vi "Begin.vi"(11 "Image Size":T1=enum."160x120") -> (0 "error out":errorcluster)   [LabVIEW 2012]
doc: "Called before other user functions, this VI is expected to open initial I/O refnums, load in file data, and do all program initialization. Notice that the <B>error out</B> terminal is simply used for data flow. Wiring it to other structures or subVIs ensures that this VI runs first."
uses:
  <vilib>/Rock Robotics/WPI/Camera/WPI_CameraImageSize.ctl
  <vilib>/Rock Robotics/SystemInterfaces/DIO/FPGA_DIOPWMChannel.ctl
  <vilib>/Rock Robotics/WPI/Camera/WPI_CameraWhite Balance Values.ctl
  <vilib>/Rock Robotics/WPI/Camera/WPI_CameraExposure Values.ctl
  <vilib>/Rock Robotics/WPI/Camera/WPI_CameraFrameRate.ctl
  <vilib>/Rock Robotics/WPI/DriverStation/WPI_DriverStationRobotMode2.ctl
  <vilib>/Rock Robotics/WPI/Joystick/WPI_JoystickDeviceEnum.ctl
  <vilib>/Rock Robotics/WPI/Solenoid/WPI_SolenoidChannel.ctl
  <vilib>/Rock Robotics/SystemInterfaces/DIO/FPGA_DIORelayChannel.ctl
  <vilib>/Rock Robotics/SystemInterfaces/DIO/FPGA_DIOChannel.ctl
  <vilib>/Rock Robotics/WPI/SafetyOutput/WPI_SafetyOutputConfigMenu.ctl
  <vilib>/Rock Robotics/WPI/RobotDrive/WPI_RobotDriveOpen2MotorWithJaguar.vi
  Robot Global Data.vi
  <vilib>/Rock Robotics/WPI/MotorControl/WPI_MotorControlOpen Jaguar.vi
  <vilib>/Rock Robotics/WPI/Solenoid/WPI_SolenoidOpenDouble.vi
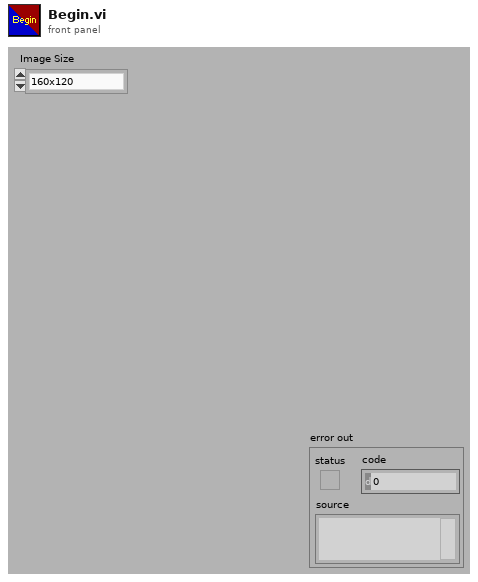
[diagram p1: front panel]
types:
  T1 = typedef "WPI_CameraImageSize.ctl" = enum16{"640x480", "320x240", "160x120"}
  T2 = typedef "WPI_SafetyOutputConfigMenu.ctl" = enum16{"Enable", "Disable"}
  T3 = typedef "FPGA_DIOPWMChannel.ctl" = enum8{"PWM 1", "PWM 2", "PWM 3", "PWM 4", "PWM 5", "PWM 6", "PWM 7", "PWM 8", "PWM 9", "PWM 10", "Invalid"}
  T4 = typedef "FPGA_DIORelayChannel.ctl" = enum8{"Relay 1", "Relay 2", "Relay 3", "Relay 4", "Relay 5", "Relay 6", "Relay 7", "Relay 8", "Invalid"}
  T5 = typedef "FPGA_DIOChannel.ctl" = enum8{"DIO 1", "DIO 2", "DIO 3", "DIO 4", "DIO 5", "DIO 6", "DIO 7", "DIO 8", "DIO 9", "DIO 10", "DIO 11", "DIO 12", "DIO 13", "DIO 14", "Invalid"}
  T6 = typedef "WPI_SolenoidChannel.ctl" = enum8{"Solenoid 1", "Solenoid 2", "Solenoid 3", "Solenoid 4", "Solenoid 5", "Solenoid 6", "Solenoid 7", "Solenoid 8", "Invalid"}
  T7 = typedef "WPI_JoystickDeviceEnum.ctl" = enum16{"USB 1", "USB 2", "USB 3", "USB 4", "Kinect 1", "Kinect 2"}
  T8 = typedef "WPI_DriverStationRobotMode2.ctl" = enum16{"Autonomous Disabled", "Autonomous Enabled", "Teleop Disabled", "Teleop Enabled", "Timeout", "Finish", "Test Disabled", "Test Enabled"}
  T9 = typedef "WPI_CameraFrameRate.ctl" = u32
  T10 = typedef "WPI_CameraExposure Values.ctl" = enum16{"Auto", "Flicker-free 50 Hz", "Flicker-free 60 Hz", "Hold current"}
  T11 = typedef "WPI_CameraWhite Balance Values.ctl" = enum16{"Auto", "Fixed indoor", "Fixed outdoor 1", "Fixed outdoor 2", "Fixed fluorescent 1", "Fixed fluorescent 2", "Hold current"}
  T12 = typedef "WPI_DigitalInputDevRef.ctl" = cluster{"DevStatus":errorcluster, "DIO Channel":T5, "Digital Module":T13}
  T13 = typedef "FPGA_TypedefDigitalModule.ctl" = enum16{"Digital Module 1", "Digital Module 2"}
  T14 = typedef "WPI_SolenoidDevRef.ctl" = cluster{"DevStatus":errorcluster, "Solenoid Module":T15, "Forward Solenoid Channel":T6, "Reverse Solenoid Channel":T6}
  T15 = typedef "FPGA_TypedefSolenoidModule.ctl" = enum16{"Solenoid Module 1", "Solenoid Module 2"}
  T16 = typedef "WPI_CameraDevRef.ctl" = cluster{"Camera Address":string, "CameraStatus":errorcluster, "Acquire Image Notifier":refnum<notifier>}
  T17 = typedef "WPI_JoystickDevRef.ctl" = cluster{"Device":T7}
  T18 = typedef "WPI_RobotDriveDevRef.ctl" = cluster{"DevStatus":errorcluster, "Motors[]":T19[], "Square Inputs":bool, "Max Output":dbl, "Isochronous":bool}
  T19 = typedef "WPI_MotorControlDeviceRef.ctl" = cluster{"DeviceStatus":errorcluster, "Type":enum16{"PWM", "CAN"}, "PWM":cluster{"Digital Module":T13, "PWM Channel":T3, "DeadBand":T20}, "CAN":cluster{"Device Number":u8, "Control Mode":T21, "Semaphore":T22, "Max Vout":dbl}, "Invert":bool, "TransformRef":T23, "InvTransformRef":T23}
  T20 = typedef "WPI_PWMDeadband.ctl" = cluster{"Name":string, "maxPositivePwm":i32, "minPositivePwm":i32, "centerPwm":i32, "maxNegativePwm":i32, "minNegativePwm":i32, "angularRange":u16}
  T21 = typedef "WPI_CANJaguar_ControlMode.ctl" = enum8{"Percent VBus", "Current", "Speed", "Position", "Voltage"}
  T22 = typedef "Semaphore RefNum" = refnum<k1>
  T23 = typedef "WPI_PWMTransform_ConPane.ctl" = refnum<vi>
  T24 = typedef "WPI_RelayDevRef.ctl" = cluster{"DevStatus":errorcluster, "Relay Channel":T4, "Digital Module":T13, "Relay Direction":T25}
  T25 = typedef "WPI_RelayDirection.ctl" = enum16{"Both directions", "Forward only", "Reverse only"}
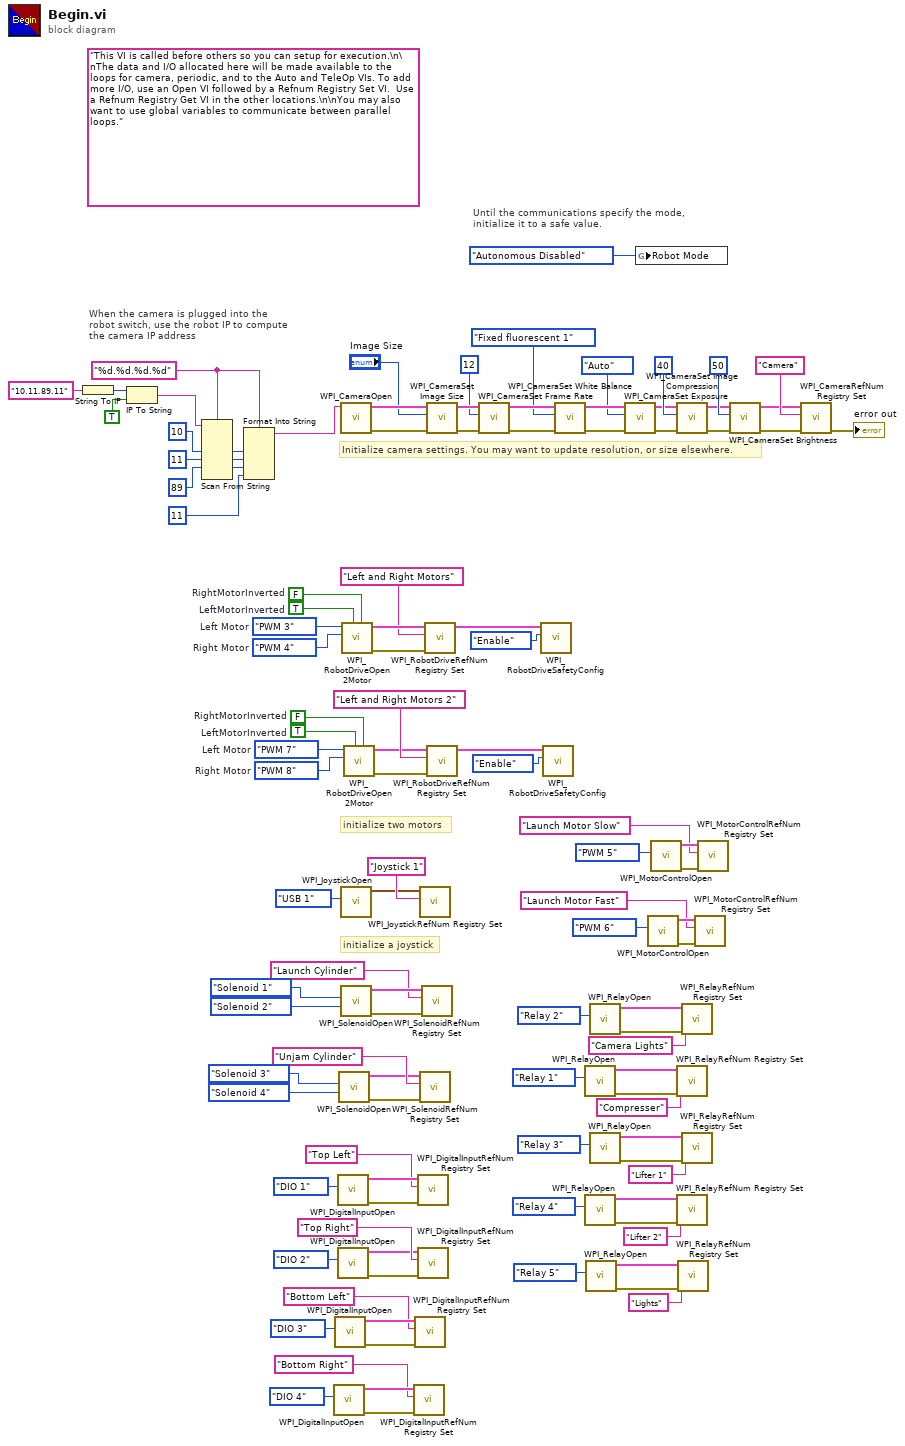
[diagram p0: block diagram]
diagram:
  w7 = FPGA_DIOPWMChannel."PWM 8"  # Right Motor
  w6 = FPGA_DIOPWMChannel."PWM 7"  # Left Motor
  w2 = TRUE  # LeftMotorInverted
  w1 = FALSE  # RightMotorInverted
  w76 = "%d.%d.%d.%d" ("format string")
  (unwired) "This VI is called before others so you can setup for execution.\n\nThe data and I/O allocated here will be made available to the loops for camera, periodic, and to the Auto and TeleOp VIs. To add more I/O, use an Open VI followed by a Refnum Registry Set VI.  Use a Refnum Registry Get VI in the other locations.\n\nYou may also want to use global variables to communicate between parallel loops."
  w87 = FPGA_DIOPWMChannel."PWM 4"  # Right Motor
  w88 = FPGA_DIOPWMChannel."PWM 3"  # Left Motor
  w110 = TRUE  # LeftMotorInverted
  w111 = FALSE  # RightMotorInverted
  # "initialize a joystick"
  # "Until the communications specify the mode,\ninitialize it to a safe value."
  # "When the camera is plugged into the\nrobot switch, use the robot IP to compute\nthe camera IP address"
  # "initialize two motors"
  # "Initialize camera settings. You may want to update resolution, or size elsewhere."
  n1 = String To IP(1:"10.11.89.11" ("name")) -> (0:w83:u32)
  n2 = IP To String(1:TRUE ("dot notation? (F)"), 2:w83) -> (0:w81:string)
  n3 = Scan From String(format string=w76, input string=w81, default 1=10 ("default value 1"), default 2=11 ("default value 2"), default 3=89 ("default value 3")) -> (output 1=w80:i32, output 2=w79:i32, output 3=w78:i32)  [unwired: 4 in, 3 out]
  n4 = Format Into String(format string=w76, w80, w79, w78, 11 ("Compression")) -> (resulting string=w72:string)  [unwired: 2 in, 1 out]
  n5 = call <vilib>:"WPI_DigitalInputOpen.vi"("DIO Channel"=FPGA_DIOChannel."DIO 4") -> ("error out"=w16:errorcluster, "DigitalInputDevRef"=w17:T12)  [unwired: 9 in]
  n6 = call <vilib>:"WPI_DigitalInputOpen.vi"("DIO Channel"=FPGA_DIOChannel."DIO 3") -> ("error out"=w21:errorcluster, "DigitalInputDevRef"=w20:T12)  [unwired: 9 in]
  n7 = call <vilib>:"WPI_DigitalInputOpen.vi"("DIO Channel"=FPGA_DIOChannel."DIO 1") -> ("error out"=w29:errorcluster, "DigitalInputDevRef"=w28:T12)  [unwired: 9 in]
  n8 = call <vilib>:"WPI_DigitalInputOpen.vi"("DIO Channel"=FPGA_DIOChannel."DIO 2") -> ("error out"=w22:errorcluster, "DigitalInputDevRef"=w23:T12)  [unwired: 9 in]
  n9 = call-poly <vilib>:"WPI_SolenoidOpen.vi"("Reverse Solenoid Channel"=WPI_SolenoidChannel."Solenoid 4", "Forward Solenoid Channel"=WPI_SolenoidChannel."Solenoid 3") -> ("error out"=w42:errorcluster, "SolenoidDevRef"=w43:T14)  [unwired: 8 in]
  n10 = call <vilib>:"WPI_CameraOpen.vi"("Camera Address"=w72) -> ("error out"=w97:errorcluster, "CameraDevRef"=w98:T16)  [unwired: 1 in, 8 out]
  n11 = call <vilib>:"WPI_JoystickOpen.vi"("JoystickDevice"=WPI_JoystickDeviceEnum."USB 1") -> ("JoystickDevRef"=w70:T17)  [unwired: 10 in]
  n12 = call-poly <vilib>:"WPI_SolenoidOpen.vi"("Reverse Solenoid Channel"=WPI_SolenoidChannel."Solenoid 2", "Forward Solenoid Channel"=WPI_SolenoidChannel."Solenoid 1") -> ("error out"=w55:errorcluster, "SolenoidDevRef"=w54:T14)  [unwired: 8 in]
  n13 = call-poly <vilib>:"WPI_RobotDriveOpen2Motor.vi"("Right Motor Inverted"=w111, "Left Motor Inverted"=w110, "Right Motor"=w87, "Left Motor"=w88) -> ("error out"=w106:errorcluster, "RobotDriveDevRef"=w108:T18)  [unwired: 1 in, 5 out]
  n14 = call-poly <vilib>:"WPI_RobotDriveOpen2Motor.vi"("Right Motor Inverted"=w1, "Left Motor Inverted"=w2, "Right Motor"=w7, "Left Motor"=w6) -> ("error out"=w5:errorcluster, "RobotDriveDevRef"=w3:T18)  [unwired: 1 in, 5 out]
  n15 = call <vilib>:"WPI_DigitalInputRefNum Registry Set.vi"("error in (no error)"=w16, "refnum name"="Bottom Right", "DigitalInputDevRef"=w17) -> ()  [unwired: 7 in, 2 out]
  n16 = call <vilib>:"WPI_DigitalInputRefNum Registry Set.vi"("error in (no error)"=w21, "refnum name"="Bottom Left", "DigitalInputDevRef"=w20) -> ()  [unwired: 7 in, 2 out]
  n17 = call <vilib>:"WPI_DigitalInputRefNum Registry Set.vi"("error in (no error)"=w29, "refnum name"="Top Left", "DigitalInputDevRef"=w28) -> ()  [unwired: 7 in, 2 out]
  n18 = call <vilib>:"WPI_DigitalInputRefNum Registry Set.vi"("error in (no error)"=w22, "refnum name"="Top Right", "DigitalInputDevRef"=w23) -> ()  [unwired: 7 in, 2 out]
  n19 = call <vilib>:"WPI_JoystickRefNum Registry Set.vi"("refnum name"="Joystick 1", "JoystickDevRef"=w70) -> ()  [unwired: 8 in, 2 out]
  n20 = call <vilib>:"WPI_SolenoidRefNum Registry Set.vi"("error in (no error)"=w42, "refnum name"="Unjam Cylinder", "SolenoidDevRef"=w43) -> ()  [unwired: 7 in, 2 out]
  n21 = call <vilib>:"WPI_SolenoidRefNum Registry Set.vi"("error in (no error)"=w55, "refnum name"="Launch Cylinder", "SolenoidDevRef"=w54) -> ()  [unwired: 7 in, 2 out]
  n22 = call <vilib>:"WPI_RobotDriveRefNum Registry Set.vi"("error in (no error)"=w106, "refnum name"="Left and Right Motors", "RobotDriveDevRef"=w108) -> ("RobotDriveDevRef"=w75:T18)  [unwired: 8 out]
  n23 = call <vilib>:"WPI_CameraSet Image Size.vi"("error in (no error)"=w97, "Image Size"="Image Size", "CameraDevRef"=w98) -> ("error out"=w96:errorcluster, "CameraDevRef Out"=w99:T16)  [unwired: 7 out]
  n24 = call <vilib>:"WPI_RobotDriveRefNum Registry Set.vi"("error in (no error)"=w5, "refnum name"="Left and Right Motors 2", "RobotDriveDevRef"=w3) -> ("RobotDriveDevRef"=w8:T18)  [unwired: 8 out]
  n25 = call <vilib>:"WPI_CameraSet Frame Rate.vi"("error in (no error)"=w96, "Frame Rate (fps)"=T9 12, "CameraDevRef"=w99) -> ("error out"=w95:errorcluster, "CameraDevRef Out"=w101:T16)  [unwired: 7 out]
  n26 = call <vilib>:"WPI_RobotDriveSafetyConfig.vi"("mode"=WPI_SafetyOutputConfigMenu."Enable", "RobotDriveDevRef"=w75) -> ()  [unwired: 8 in, 2 out]
  n27 = call <vilib>:"WPI_RobotDriveSafetyConfig.vi"("mode"=WPI_SafetyOutputConfigMenu."Enable", "RobotDriveDevRef"=w8) -> ()  [unwired: 8 in, 2 out]
  n28 = call <vilib>:"WPI_CameraSet White Balance.vi"("error in (no error)"=w95, "White Balance"=WPI_CameraWhite_Balance_Values."Fixed fluorescent 1", "CameraDevRef"=w101) -> ("error out"=w94:errorcluster, "CameraDevRef Out"=w100:T16)  [unwired: 7 out]
  n29 = call <vilib>:"WPI_RelayOpen.vi"("Relay Channel"=FPGA_DIORelayChannel."Relay 1") -> ("error out"=w38:errorcluster, "RelayDevRef"=w39:T24)  [unwired: 9 in]
  n30 = call <vilib>:"WPI_RelayOpen.vi"("Relay Channel"=FPGA_DIORelayChannel."Relay 4") -> ("error out"=w37:errorcluster, "RelayDevRef"=w36:T24)  [unwired: 9 in]
  n31 = call <vilib>:"WPI_RelayOpen.vi"("Relay Channel"=FPGA_DIORelayChannel."Relay 5") -> ("error out"=w11:errorcluster, "RelayDevRef"=w12:T24)  [unwired: 9 in]
  n32 = call <vilib>:"WPI_RelayOpen.vi"("Relay Channel"=FPGA_DIORelayChannel."Relay 2") -> ("error out"=w50:errorcluster, "RelayDevRef"=w49:T24)  [unwired: 9 in]
  n33 = call <vilib>:"WPI_RelayOpen.vi"("Relay Channel"=FPGA_DIORelayChannel."Relay 3") -> ("error out"=w30:errorcluster, "RelayDevRef"=w31:T24)  [unwired: 9 in]
  n34 = call <vilib>:"WPI_CameraSet Exposure.vi"("error in (no error)"=w94, "Exposure"=WPI_CameraExposure_Values."Auto", "CameraDevRef"=w100) -> ("error out"=w93:errorcluster, "CameraDevRef Out"=w103:T16)  [unwired: 7 out]
  n35 = global write "Robot Global Data.vi" "Robot Mode"(WPI_DriverStationRobotMode2."Autonomous Disabled" ("Robot Mode")) -> ()
  n36 = call-poly <vilib>:"WPI_MotorControlOpen.vi"("PWM Channel"=FPGA_DIOPWMChannel."PWM 6") -> ("error out"=w58:errorcluster, "MotorControlDeviceRef"=w59:T19)  [unwired: 9 in]
  n37 = call-poly <vilib>:"WPI_MotorControlOpen.vi"("PWM Channel"=FPGA_DIOPWMChannel."PWM 5") -> ("error out"=w66:errorcluster, "MotorControlDeviceRef"=w67:T19)  [unwired: 9 in]
  n38 = call <vilib>:"WPI_CameraSet Image Compression.vi"("error in (no error)"=w93, "Compression"=40, "CameraDevRef"=w103) -> ("error out"=w92:errorcluster, "CameraDevRef Out"=w102:T16)  [unwired: 7 out]
  n39 = call <vilib>:"WPI_RelayRefNum Registry Set.vi"("error in (no error)"=w38, "refnum name"="Compresser", "RelayDevRef"=w39) -> ()  [unwired: 7 in, 2 out]
  n40 = call <vilib>:"WPI_RelayRefNum Registry Set.vi"("error in (no error)"=w37, "refnum name"="Lifter 2", "RelayDevRef"=w36) -> ()  [unwired: 7 in, 2 out]
  n41 = call <vilib>:"WPI_RelayRefNum Registry Set.vi"("error in (no error)"=w11, "refnum name"="Lights", "RelayDevRef"=w12) -> ()  [unwired: 7 in, 2 out]
  n42 = call <vilib>:"WPI_RelayRefNum Registry Set.vi"("error in (no error)"=w50, "refnum name"="Camera Lights", "RelayDevRef"=w49) -> ()  [unwired: 7 in, 2 out]
  n43 = call <vilib>:"WPI_RelayRefNum Registry Set.vi"("error in (no error)"=w30, "refnum name"="Lifter 1", "RelayDevRef"=w31) -> ()  [unwired: 7 in, 2 out]
  n44 = call <vilib>:"WPI_MotorControlRefNum Registry Set.vi"("error in (no error)"=w58, "refnum name"="Launch Motor Fast", "MotorControlDevRef"=w59) -> ()  [unwired: 7 in, 2 out]
  n45 = call <vilib>:"WPI_MotorControlRefNum Registry Set.vi"("error in (no error)"=w66, "refnum name"="Launch Motor Slow", "MotorControlDevRef"=w67) -> ()  [unwired: 7 in, 2 out]
  n46 = call <vilib>:"WPI_CameraSet Brightness.vi"("error in (no error)"=w92, "Brightness"=50, "CameraDevRef"=w102) -> ("error out"=w90:errorcluster, "CameraDevRef Out"=w91:T16)  [unwired: 7 out]
  n47 = call <vilib>:"WPI_CameraRefNum Registry Set.vi"("error in (no error)"=w90, "refnum name"="Camera", "CameraDevRef"=w91) -> ("error out"=→"error out":errorcluster)  [unwired: 8 out]
